vi "CMWinitallTypes.vi"(8 "error in":errorcluster, 10 "Data Type":string, 11 "URL":string="VAC.VGHA_41677/PR") -> (0 "error out":errorcluster, 3 "CMWout":refnum<class "CMWSubscribe.lvclass">)   [LabVIEW 2014]
uses:
  <userlib>/_RADE/RIO/CMW/classes/CMWSubscribe/CMWSubscribe.lvclass
  <userlib>/_RADE/RIO/CMW/classes/CMWSubscribe/openCMWSubscribe.vi
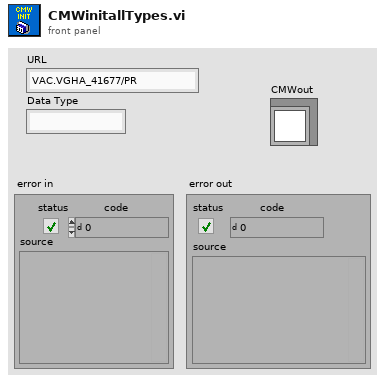
[diagram p1: front panel]
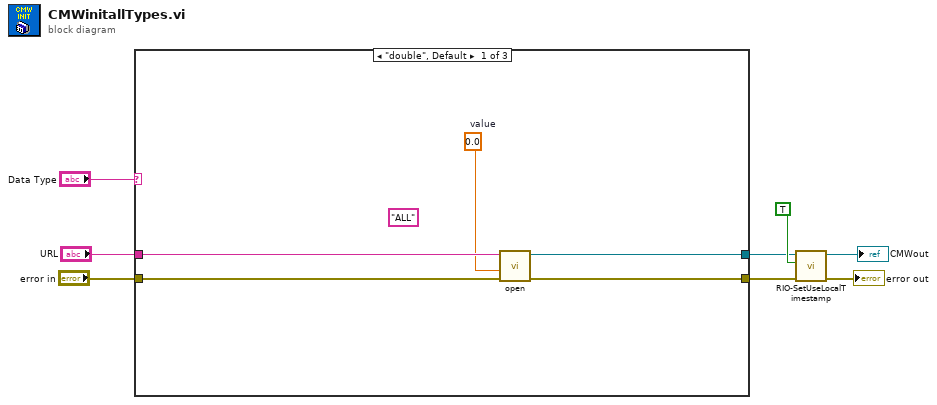
[diagram p0: block diagram]
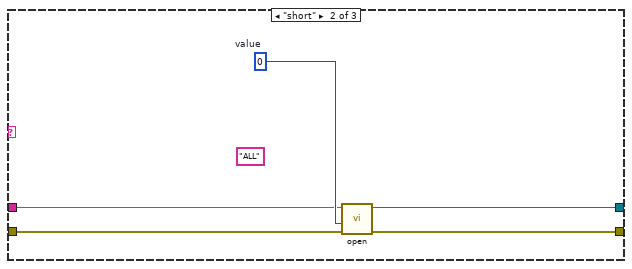
[diagram p2: hidden frame]
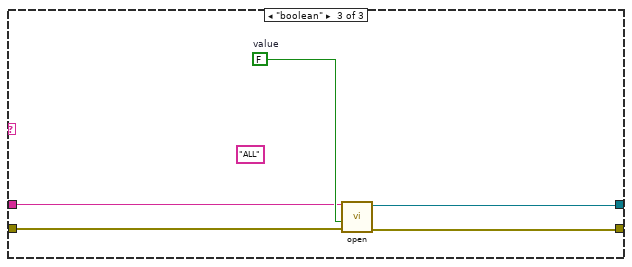
[diagram p3: hidden frame]
diagram:
  n1 = case shown="\"double\", Default" "Data Type" {
    tunnel: "error in" -> [w12 w18 w21]
    tunnel: [w11 w14 w22] -> w4
    tunnel: "URL" -> [w13 w16 w19]
    tunnel: [w10 w15 w20] -> w2
    frame "double", Default {
      w9 = sgl 0.0  # value
      (unwired) "ALL" ("Cycle")
      n2 = call-poly <userlib>:"open.vi"("error in (no error)"=w12, "Data type"=w9, "URL"=w13) -> ("error out"=w11:errorcluster, "Object out"=w10:refnum<class "CMWSubscribe.lvclass">)  [unwired: 7 in]
    }
    frame "short" {
      w17 = i16 0  # value
      (unwired) "ALL" ("Cycle")
      n3 = call-poly <userlib>:"open.vi"("error in (no error)"=w18, "Data type"=w17, "URL"=w16) -> ("error out"=w14:errorcluster, "Object out"=w15:refnum<class "CMWSubscribe.lvclass">)  [unwired: 7 in]
    }
    frame "boolean" {
      w23 = FALSE  # value
      (unwired) "ALL" ("Cycle")
      n4 = call-poly <userlib>:"open.vi"("error in (no error)"=w21, "Data type"=w23, "URL"=w19) -> ("error out"=w22:errorcluster, "Object out"=w20:refnum<class "CMWSubscribe.lvclass">)  [unwired: 7 in]
    }
  }
  n5 = call-dynamic "RIO-SetUseLocalTimestamp.vi"("error in (no error)"=w4, "Use Local Timestamp?"=TRUE, "CMWBase in"=w2) -> ("error out"=→"error out":errorcluster, "CMWBase out"=→"CMWout":refnum<class "CMWSubscribe.lvclass">)  [unwired: 7 in]
